vi "Check For Winner Board.vi"(8 "Matrixes Status In":bool[][][](array[boolean]), 10 "Turn Number":i32, 11 "Boards":i32[][][](array[numeric])) -> (0 "Matrixes Status Out":bool[][][](array[boolean]), 1 "Winner Board Status":bool[][](array[boolean]), 2 "Winner Board":i32[][](array[numeric]), 3 "Winner Found?":bool)   [LabVIEW 2019, in "Day 4.lvlib"]
uses:
  Day 4.lvlib
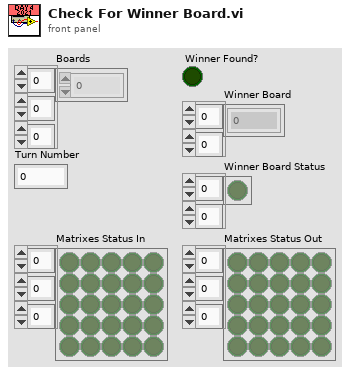
[diagram p1: front panel]
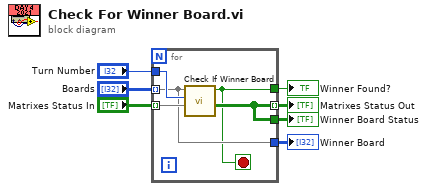
[diagram p0: block diagram]
diagram:
  n1 = for {
    tunnel: "Boards" -> [w9] mode=indexing
    tunnel: "Turn Number" -> [w12]
    tunnel: [w10] -> w5 mode=indexing
    tunnel: "Matrixes Status In" -> [w11] mode=indexing
    tunnel: [w10] -> w3
    tunnel: [w9] -> w2
    tunnel: [w8] -> w1
    stop <- w8 stop-if-true
    n2 = call "Check If Winner Board.vi"("Matriz Status In"=w11, "Turn Number"=w12, "Boards"=w9) -> ("Matriz Status Out"=w10:bool[][], "Winner?"=w8:bool)  [unwired: 7 in]
  }
  "Matrixes Status Out" <- w5
  "Winner Board Status" <- w3
  "Winner Board" <- w2
  "Winner Found?" <- w1
